vi "frog_newport_final.vi"() -> ()   [LabVIEW 2016]
uses:
  <instrlib>/Ocean Optics 2000 4000/Ocean Optics 2000 4000.lvlib
  Downloads/ESP301_LabVIEW_Drivers/Newport ESP301/Newport ESP301.lvlib
panel:
  in  "Axis":i32=3 min=1 max=3
  in  "error in (no error)":errorcluster
  in  "Reset (False)":bool
  in  "ID Query (True)":bool=TRUE
  in  "VISA resource name Translation Stage":refnum<visa-resource-name>="COM3"
  in  "Integration Time (6000us)":u32=6000
  in  "Average #":i32=5
  out "Spectral Waveform":cluster{dbl[], dbl[]}(graph)
  out "0.5*Max intens":dbl=4438.0
  in  "Final Position, mm":ext=21.35
  out "Pulse":dbl[][](graph)
  in  "Start FROG":bool
  in  "Enable Strobe (Disabled)":bool
  in  "VISA resource name":refnum<visa-resource-name>="USB0::0x2457::0x1012::NI-VISA-10001::RAW"
  in  "Initial Position, mm":ext=21.299999999999999999
  in  "Step Size, mm":ext=0.0001
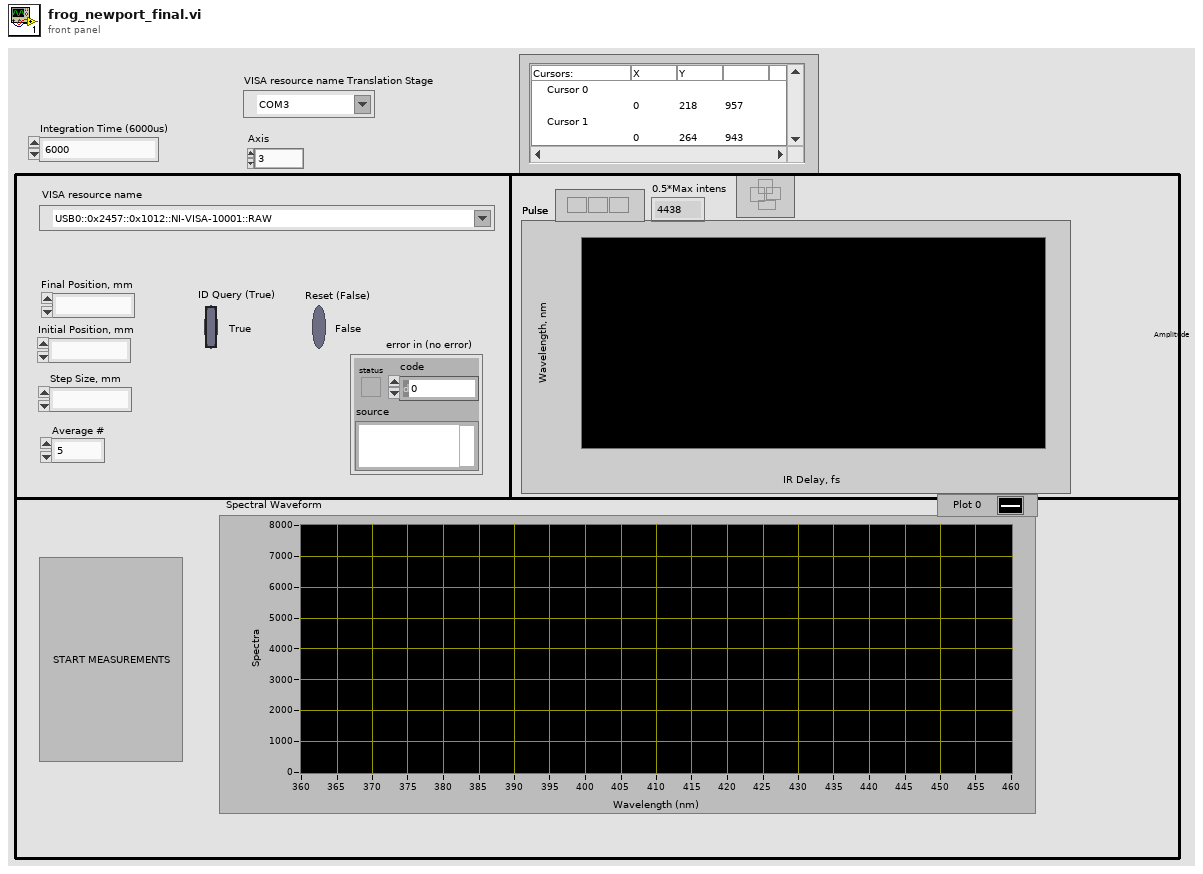
[diagram p1: front panel]
types:
  T1 = cluster{"Wavelength (nm)":dbl[], "Spectrum by Pixel Number":dbl[]}
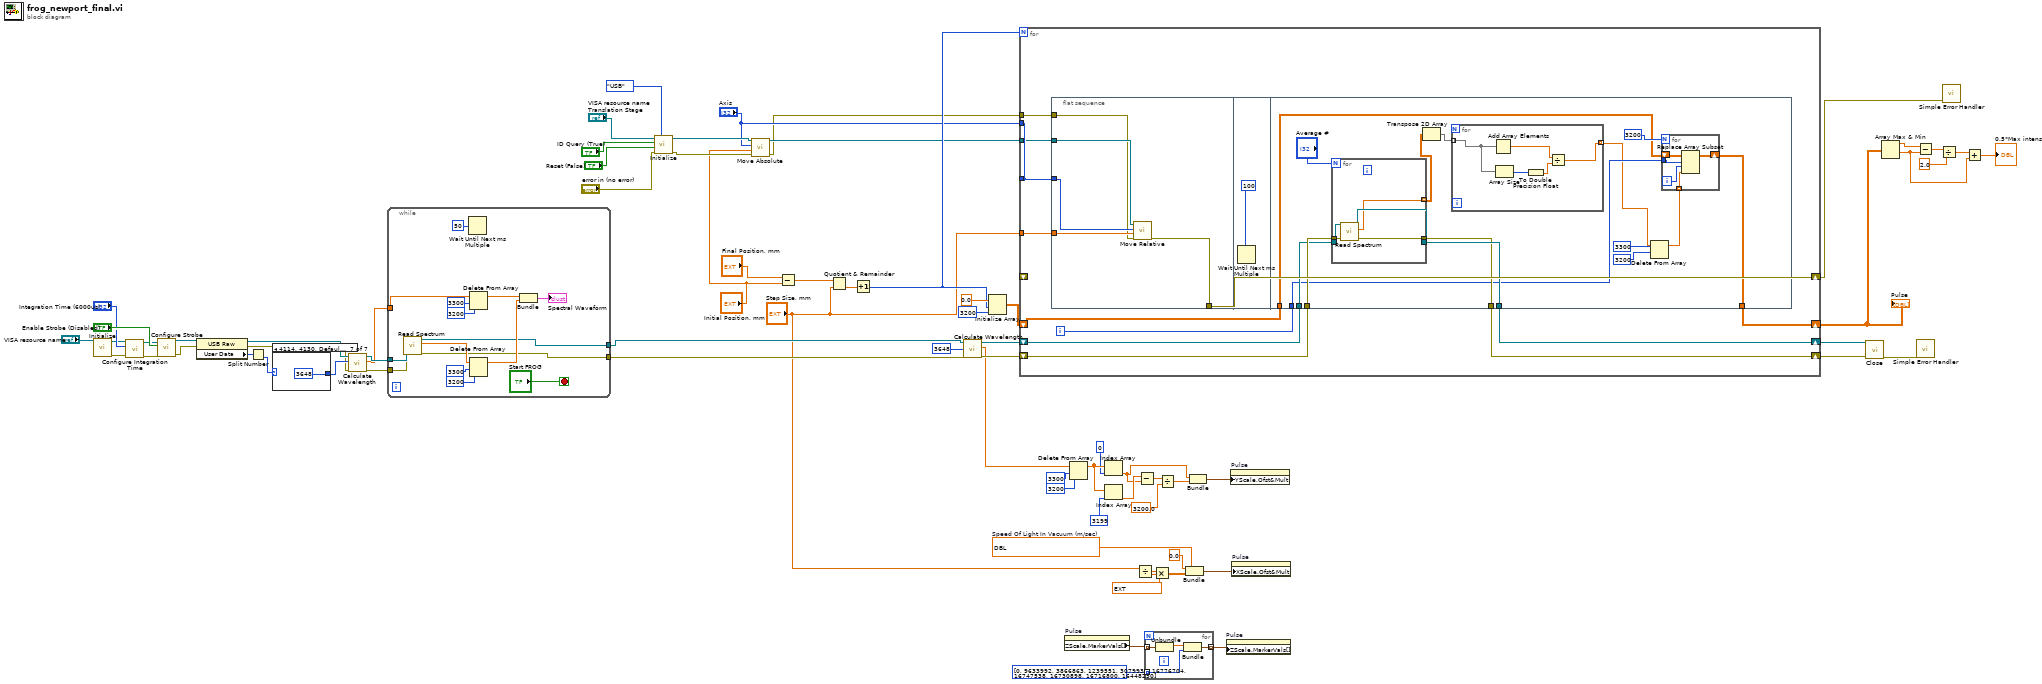
[diagram p0: block diagram]
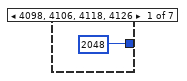
[diagram p2: hidden frame]
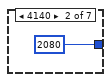
[diagram p3: hidden frame]
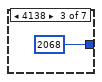
[diagram p4: hidden frame]
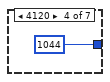
[diagram p5: hidden frame]
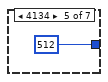
[diagram p6: hidden frame]
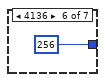
[diagram p7: hidden frame]
diagram:
  w62 = ext[unit] 299792458.0  # Speed Of Light In Vacuum (m/sec)
  n1 = call <instrlib>:"Initialize.vi"("VISA resource name"="VISA resource name") -> ("error out"=w16:errorcluster, "VISA resource name out"=w17:refnum<visa-resource-name>)  [unwired: 2 in, 7 out]
  n2 = call <instrlib>:"Configure Integration Time.vi"("error in (no error)"=w16, "Integration Time (6000)"="Integration Time (6000us)", "VISA resource name"=w17) -> ("error out"=w15:errorcluster, "VISA resource name out"=w14:refnum<visa-resource-name>)  [unwired: 7 out]
  n3 = call <instrlib>:"Configure Strobe.vi"("error in (no error)"=w15, "Enable Strobe (Disabled)"="Enable Strobe (Disabled)", "VISA resource name"=w14) -> ("error out"=w35:errorcluster, "VISA resource name out"=w34:refnum<visa-resource-name>)  [unwired: 7 out]
  n4 = property class="USB Raw"(reference=w34, error in=w35) -> (reference out=w32:refnum<visa-resource-name>, error out=w31:errorcluster, "User Data"=w53:u32)
  n5 = Split Number(x=w53) -> (lo(x)=w52:u16)  [unwired: 1 out]
  n6 = case shown="4114, 4130, Default" w52 {
    tunnel: [2048 ("Number of Pixels (3840)") 2080 ("Number of Pixels (3840)") 2068 ("Number of Pixels (3840)") 1044 ("Number of Pixels (3840)") 512 ("Number of Pixels (3840)") 256 ("Number of Pixels (3840)") 3648 ("Number of Pixels (3840)")] -> w33
    frame 4098, 4106, 4118, 4126 {
    }
    frame 4140 {
    }
    frame 4138 {
    }
    frame 4120 {
    }
    frame 4134 {
    }
    frame 4136 {
    }
    frame 4114, 4130, Default {
    }
  }
  n7 = call <instrlib>:"Calculate Wavelength.vi"("error in (no error)"=w31, "Number of Pixels (3648)"=w33, "VISA resource name"=w32) -> ("error out"=w29:errorcluster, "Wavelength (nm)"=w19:dbl[], "VISA resource name out"=w30:refnum<visa-resource-name>)  [unwired: 6 out]
  n8 = while {
    tunnel: w30 -> [w88]
    tunnel: w29 -> [w87]
    tunnel: w19 -> [w86]
    tunnel: [w82] -> w27
    tunnel: [w81] -> w26
    stop <- "Start FROG" stop-if-true
    n9 = call <instrlib>:"Read Spectrum.vi"("error in (no error)"=w87, "VISA resource name"=w88) -> ("error out"=w81:errorcluster, "Spectrum by Pixel Number"=w84:dbl[], "VISA resource name out"=w82:refnum<visa-resource-name>)  [unwired: 6 in, 1 out]
    n10 = Wait Until Next ms Multiple(millisecond multiple=u32 50) -> ()  [unwired: 1 out]
    n11 = Delete From Array(array=w84, length=3300, index=3200) -> (array with subset deleted=w85:dbl[])  [unwired: 1 out]
    n12 = Delete From Array(array=w86, length=3300, index=3200) -> (array with subset deleted=w89:dbl[])  [unwired: 1 out]
    n13 = Bundle("Wavelength (nm)"=w89, "Spectrum by Pixel Number"=w85) -> (→"Spectral Waveform":T1)  [unwired: 1 out]
  }
  n14 = call <instrlib>:"Initialize.vi"("VISA resource name"="VISA resource name Translation Stage", "ID Query (True)"="ID Query (True)", "Reset (False)"="Reset (False)", "error in (no error)"="error in (no error)", "Serial Link (RS232)"=enum16{"RS232", "USB"}."USB") -> ("VISA resource name out"=w7:refnum<visa-resource-name>, "error out"=w8:errorcluster)  [unwired: 4 in]
  n15 = call "Move Absolute.vi"("error in (no error)"=w8, "Position (0 units)"="Initial Position, mm", "Axis (1)"="Axis", "VISA resource name"=w7) -> ("error out"=w1:errorcluster, "VISA resource name out"=w4:refnum<visa-resource-name>)  [unwired: 2 in]
  n16 = Subtract(x="Final Position, mm", y="Initial Position, mm") -> (x-y=w50:ext)
  n17 = Quotient & Remainder(x=w50, y="Step Size, mm") -> (floor(x/y)=w49:ext)  [unwired: 1 out]
  n18 = Increment(x=w49) -> (x+1=w46:i32)
  n19 = call <instrlib>:"Calculate Wavelength.vi"("error in (no error)"=w26, "Number of Pixels (3648)"=3648, "VISA resource name"=w27) -> ("error out"=w24:errorcluster, "Wavelength (nm)"=w23:dbl[], "VISA resource name out"=w25:refnum<visa-resource-name>)  [unwired: 6 out]
  n20 = Initialize Array(0.0 ("element"), w46, 3200 ("dimension size")) -> (w45:dbl[][])
  n21 = for {
    N: w46 -> [_]
    tunnel: [w101] -> _
    shift-right: [w105] -> w22
    shift-left: w25 -> [w107]
    shift-right: [w104] -> w21
    shift-left: w24 -> [w106]
    shift-right: [w102] -> w44
    shift-left: w45 -> [w98]
    tunnel: "Axis" -> [w101]
    tunnel: w4 -> [w100]
    tunnel: "Step Size, mm" -> [w99]
    shift-right: [w97] -> w2
    shift-left: _ -> [_]
    tunnel: w1 -> [w96]
    i -> [w103]
    n22 = flat-sequence {
      tunnel: w101 -> [w112]
      tunnel: w100 -> [w111]
      tunnel: w99 -> [w110]
      tunnel: [w109] -> w97
      tunnel: w96 -> [w108]
      tunnel: w107 -> [w121]
      tunnel: w106 -> [w122]
      tunnel: [w119] -> w104
      tunnel: [w120] -> w105
      tunnel: w103 -> [w118]
      tunnel: w98 -> [w124]
      tunnel: [w123] -> w102
      frame #0 {
        n23 = call "Move Relative.vi"("error in (no error)"=w108, "Position (0 units)"=w110, "Axis (1)"=w112, "VISA resource name"=w111) -> ("error out"=w109:errorcluster)  [unwired: 2 in, 1 out]
      }
      frame #1 {
        n24 = Wait Until Next ms Multiple(millisecond multiple=u32 100) -> ()  [unwired: 1 out]
      }
      frame #2 {
        n25 = for {
          N: "Average #" -> [_]
          tunnel: [w134] -> w115 mode=indexing
          tunnel: w122 -> [w138]
          tunnel: [w135] -> w119
          tunnel: w121 -> [w137]
          tunnel: [w136] -> w120
          n26 = call <instrlib>:"Read Spectrum.vi"("error in (no error)"=w138, "VISA resource name"=w137) -> ("error out"=w135:errorcluster, "Spectrum by Pixel Number"=w134:dbl[], "VISA resource name out"=w136:refnum<visa-resource-name>)  [unwired: 6 in, 1 out]
        }
        n27 = Transpose 2D Array(2D array=w115) -> (transposed array=w114:dbl[][])
        n28 = for {
          tunnel: [w130] -> w116 mode=indexing
          tunnel: w114 -> [w129] mode=indexing
          n29 = Add Array Elements(numeric array=w129) -> (sum=w131:dbl)
          n30 = Array Size(array=w129) -> (size(s)=w133:i32)
          n31 = To Double Precision Float(number=w133) -> (double precision float=w132:dbl)
          n32 = Divide(x=w131, y=w132) -> (x/y=w130:dbl)
        }
        n33 = Delete From Array(array=w116, length=3200, index=3300) -> (array with subset deleted=w125:dbl[])  [unwired: 1 out]
        n34 = for {
          N: 3200 -> [_]
          shift-right: [w142] -> w123
          shift-left: w124 -> [w143]
          tunnel: w118 -> [w139]
          tunnel: w125 -> [w141] mode=indexing
          i -> [w140]
          n35 = Replace Array Subset(array=w143, new element=w141, index (row)=w139, index (col)=w140) -> (w142:dbl[][])
        }
      }
    }
  }
  "Pulse" <- w44
  n36 = property on="Pulse" class="IntGraph (strict)"() -> ("ZScale.MarkerVals[]"=w56:cluster{dbl, u32}[])  [unwired: 2 in, 2 out]
  n37 = Delete From Array(array=w23, length=3300, index=3200) -> (array with subset deleted=w71:dbl[])  [unwired: 1 out]
  n38 = Index Array(array=w71, index=0) -> (element=w63:dbl)
  n39 = Index Array(array=w71, index=3199) -> (element=w68:dbl)
  n40 = Divide(x="Step Size, mm", y=w62) -> (x/y=w61:ext)
  n41 = Subtract(x=w68, y=w63) -> (x-y=w66:dbl)
  n42 = for {
    tunnel: w56 -> [w147] mode=indexing
    tunnel: u32[] [0, 9633992, 3866863, 1239551, 3079936, 16776704, 16747538, 16730898, 16716800, 16448250] ("Custom Marker Colors 2") -> [w145] mode=indexing
    tunnel: [w144] -> w55 mode=indexing
    n43 = Unbundle(w147) -> (w146:dbl)  [unwired: 1 out]
    n44 = Bundle(w146, "Color Box"=w145) -> (w144:cluster{dbl, "Color Box":u32})  [unwired: 1 in]
  }
  n45 = Multiply(x=w61, y=ext 2000000000000.0) -> (x*y=w58:ext)
  n46 = Divide(x=w66, y=3200.0) -> (x/y=w65:dbl)
  n47 = Bundle(0.0, w58) -> (w59:cluster{dbl, ext})  [unwired: 1 in]
  n48 = Bundle(w63, w65) -> (w64:cluster{dbl, dbl})  [unwired: 1 in]
  n49 = property on="Pulse" class="IntGraph (strict)"("ZScale.MarkerVals[]"=w55) -> ()  [unwired: 2 in, 2 out]
  n50 = property on="Pulse" class="IntGraph (strict)"("YScale.Ofst&Mult"=w64) -> ()  [unwired: 2 in, 2 out]
  n51 = property on="Pulse" class="IntGraph (strict)"("XScale.Ofst&Mult"=w59) -> ()  [unwired: 2 in, 2 out]
  n52 = call <instrlib>:"Close.vi"("error in (no error)"=w21, "VISA resource name"=w22) -> ("error out"=w20:errorcluster)  [unwired: 9 out]
  n53 = Array Max & Min(array=w44) -> (max value=w43:dbl, min value=w39:dbl)  [unwired: 2 out]
  n54 = call <vilib>:"Simple Error Handler.vi"("error in (no error)"=w20) -> ()  [unwired: 1 in, 8 out]
  n55 = Subtract(x=w43, y=w39) -> (x-y=w42:dbl)
  n56 = Divide(x=w42, y=2.0) -> (x/y=w40:dbl)
  n57 = call <vilib>:"Simple Error Handler.vi"("error in (no error)"=w2) -> ()  [unwired: 1 in, 8 out]
  n58 = Add(x=w40, y=w39) -> (x+y=→"0.5*Max intens":dbl)
